vi "Volume dB.vi"(8 "error in (no error)":errorcluster, 11 "RGetInputVolume in":refnum<class "RGetInputVolume.lvclass">) -> (0 "error out":errorcluster, 2 "Volume dB":dbl, 3 "RGetInputVolume out":refnum<class "RGetInputVolume.lvclass">)   [LabVIEW 2022 SP3, in "obs-websocket-lv.lvlib" / "RGetInputVolume.lvclass"]
uses:
  RGetInputVolume.lvclass
  RGetInputVolume.lvclass/RGetInputVolume.ctl
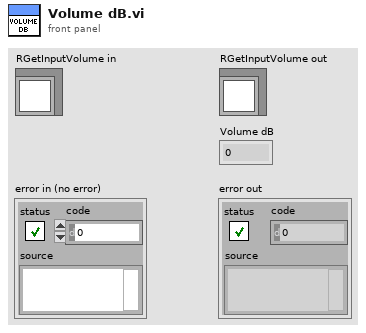
[diagram p1: front panel]
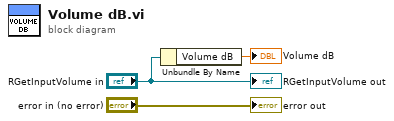
[diagram p0: block diagram]
diagram:
  n1 = Unbundle By Name("RGetInputVolume in") -> ("Volume dB"=→"Volume dB":dbl)
  "error out" <- "error in (no error)"
  "RGetInputVolume out" <- "RGetInputVolume in"
